vi "check_SN_length_.vi"(9 "min length":string, 10 "max length":string, 11 "SN in":string) -> (1 "in range?":bool, 3 "SN out":string)   [LabVIEW 2024]
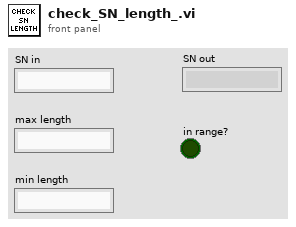
[diagram p1: front panel]
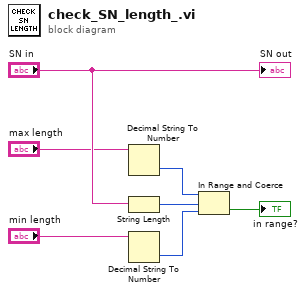
[diagram p0: block diagram]
diagram:
  n1 = Decimal String To Number(string="max length") -> (number=w3:i32)  [unwired: 2 in, 1 out]
  n2 = String Length(string="SN in") -> (length=w1:i32)
  n3 = Decimal String To Number(string="min length") -> (number=w4:i32)  [unwired: 2 in, 1 out]
  n4 = In Range and Coerce(upper limit=w3, x=w1, lower limit=w4) -> (In Range?=→"in range?":bool)  [unwired: 1 out]
  "SN out" <- "SN in"
